vi "Read Project.vi"(8 "error in (no error)":errorcluster, 11 "Parameters in":refnum<class "Parameters.lvclass">) -> (0 "error out":errorcluster, 2 "Project":T1, 3 "Parameters out":refnum<class "Parameters.lvclass">)   [LabVIEW 2023, in "Parameters.lvclass"]
uses:
  Parameters.lvclass
  Project.ctl
  Parameters.lvclass/Parameters.ctl
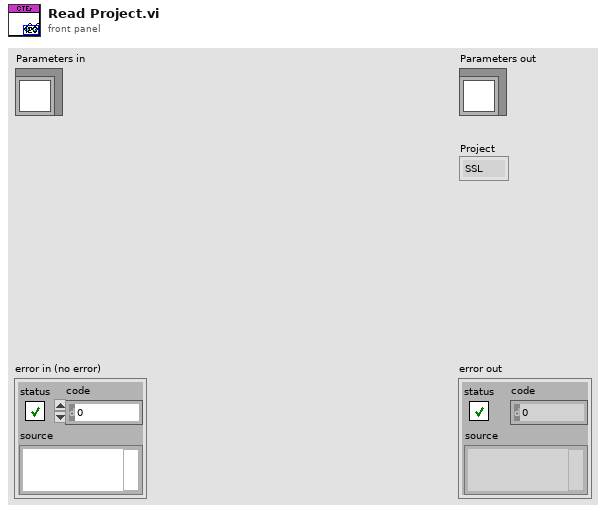
[diagram p1: front panel]
types:
  T1 = typedef "Project.ctl" = enum16{"SSL", "VSS"}
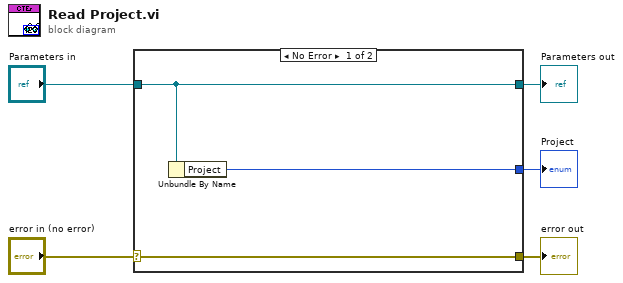
[diagram p0: block diagram]
diagram:
  n1 = case shown="No Error" "error in (no error)" {
    selector: "error in (no error)" -> [w8 w9]
    tunnel: [w8 w9] -> w4
    tunnel: [w7 w10] -> w2
    tunnel: "Parameters in" -> [w7 w10]
    tunnel: [w6 _] -> w1
    frame No Error {
      n2 = Unbundle By Name(w7) -> ("Project"=w6:T1)
    }
    frame Error {
    }
  }
  "error out" <- w4
  "Parameters out" <- w2
  "Project" <- w1
